vi "GUILaptop.vi"() -> ()   [LabVIEW 2016]
uses:
  Control/Fahrart.ctl
  Control/StreamCluster.ctl
  Control/GUICluster.ctl
panel:
  in  "Automatisch":bool
  out "stop 2":bool
  in  "Start":bool
  in  "Fahrzustand":T1
  in  "stop":bool
  in  "Geschwindigkeit multiplikator":dbl(knob)=0.039196582802747515 scale=0.0..1.0
  out "Linefollow-Array":bool[](array[boolean])
  out "Geschwindigkeit [m/s]":dbl(knob) scale=0.0..4.5
  out "Rundenzeit":T2
  out "schräg L":dbl format="%#_3g"
  out "schräge R":dbl format="%#_3g"
  out "hinten links":dbl
  out "Leistung [W]":dbl(graph)
  out "hinten rechts":dbl
  out "rechts":dbl format="%#_3g"
  out "links":dbl format="%#_3g"
  out "gerade L":dbl format="%#_3g"
  out "gerade R":dbl format="%#_3g"
  # "Minimum"
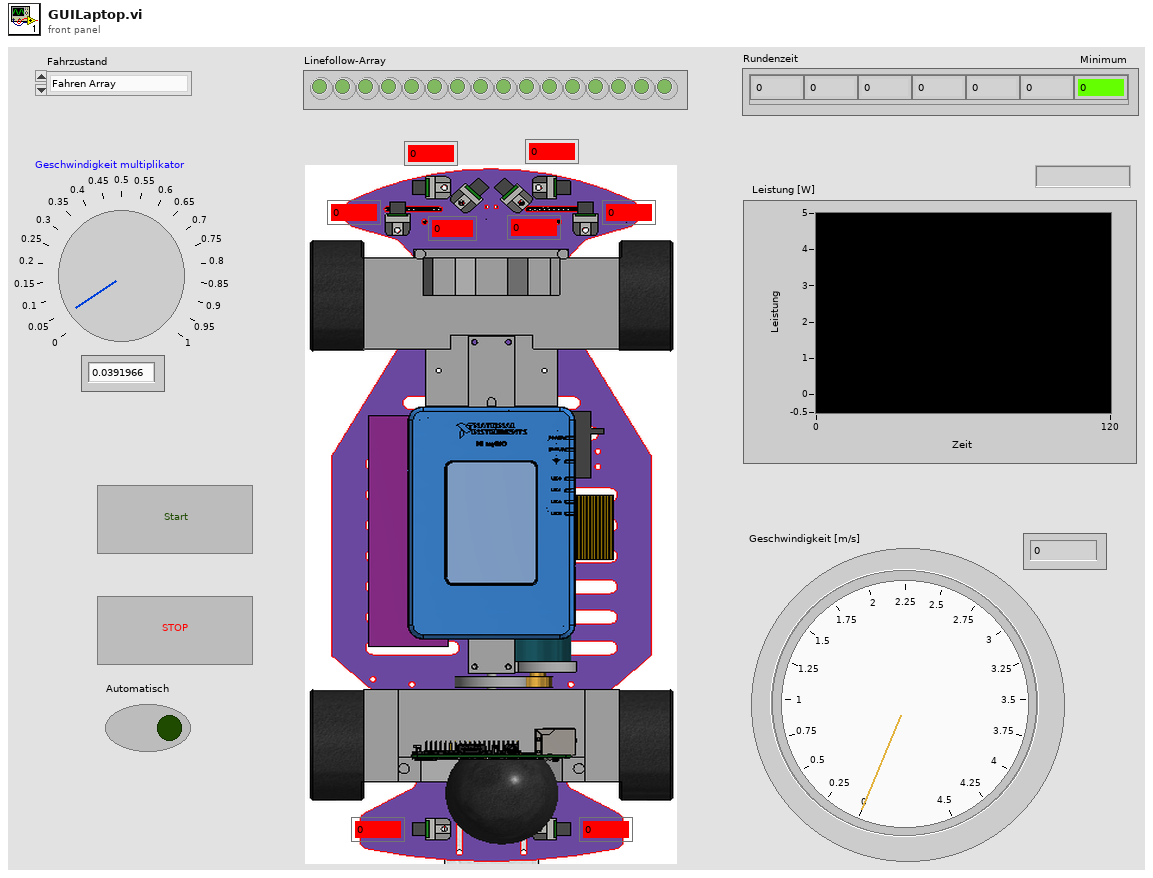
[diagram p1: front panel]
types:
  T1 = typedef "Fahrart.ctl" = enum16{"Fahren Array", "Folgen", "Überholen"}
  T2 = cluster{"Numeric":dbl, "Numeric 2":dbl, "Numeric 3":dbl, "Numeric 4":dbl, "Numeric 5":dbl, "Numeric 6":dbl, "Numeric 7":dbl}
  T3 = typedef "StreamCluster.ctl" = cluster{"IRSensoren":dbl[], "LineArray":bool[], "Rundenzeit":dbl[], "Drehzahl":dbl, "Leistung":dbl}
  T4 = typedef "GUICluster.ctl" = cluster{"Fahrart":T1, "Geschwindigkeitsmultiplikator":dbl, "Stop":bool, "Automatisch":bool}
  T5 = cluster{"Rundenzeit[0]":dbl, "Rundenzeit[1]":dbl, "Rundenzeit[2]":dbl, "Rundenzeit[3]":dbl, "Rundenzeit[4]":dbl, "Rundenzeit[5]":dbl, "Rundenzeit[6]":dbl}
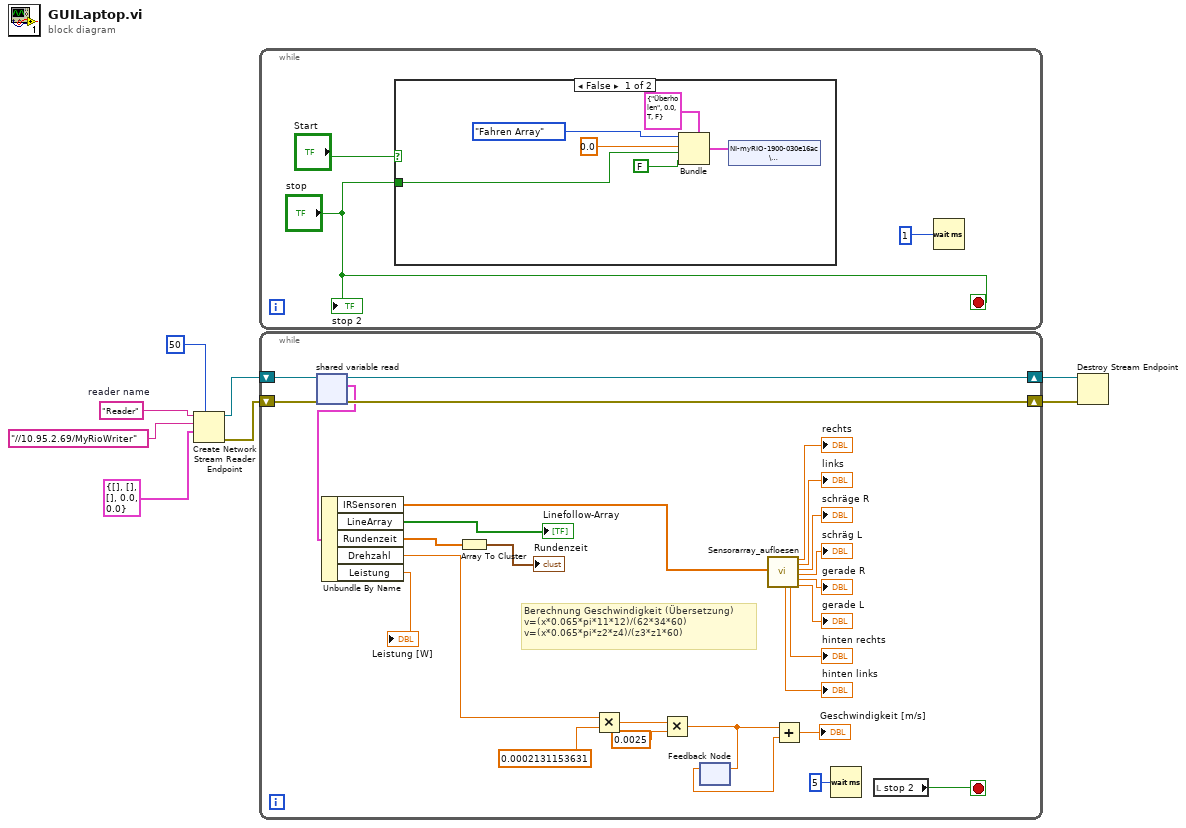
[diagram p0: block diagram]
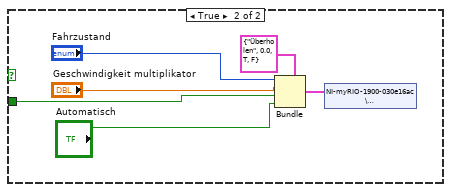
[diagram p2: hidden frame]
diagram:
  w4 = "Reader"  # reader name
  n1 = Create Network Stream Reader Endpoint(7:50 ("reader buffer size"), 9:T3 {"IRSensoren"=[], "LineArray"=[], "Rundenzeit"=[], "Drehzahl"=0.0, "Leistung"=0.0} ("Cluster"), 10:"//10.95.2.69/MyRioWriter" ("writer url"), 11:w4) -> (0:w7:errorcluster, 3:w8:refnum<k21>)  [unwired: 3 in]
  n2 = while {
    stop <- "stop" stop-if-true
    n3 = case shown="False" "Start" {
      tunnel: "stop" -> [w12 w18]
      frame False {
        n4 = Bundle(cluster=T4 {"Fahrart"=enum."Überholen", "Geschwindigkeitsmultiplikator"=0.0, "Stop"=TRUE, "Automatisch"=FALSE} ("Cluster"), "Fahrart"=Fahrart."Fahren Array" ("Enum"), "Geschwindigkeitsmultiplikator"=0.0, "Stop"=w12, "Automatisch"=FALSE ("Stop")) -> (w17:T4)
        n5 = shared-variable "NI-myRIO-1900-030e16ac\\GUICommunicationLibrary.lvlib\\GUIInput"(w17) -> ()  [unwired: 1 in, 1 out]
      }
      frame True {
        n6 = Bundle(cluster=T4 {"Fahrart"=enum."Überholen", "Geschwindigkeitsmultiplikator"=0.0, "Stop"=TRUE, "Automatisch"=FALSE} ("Cluster"), "Fahrart"="Fahrzustand", "Geschwindigkeitsmultiplikator"="Geschwindigkeit multiplikator", "Stop"=w18, "Automatisch"="Automatisch") -> (w21:T4)
        n7 = shared-variable "NI-myRIO-1900-030e16ac\\GUICommunicationLibrary.lvlib\\GUIInput"(w21) -> ()  [unwired: 1 in, 1 out]
      }
    }
    n8 = Wait (ms)(milliseconds to wait=u32 1) -> ()  [unwired: 1 out]
    "stop 2" <- "stop"
  }
  n9 = while {
    shift-right: [w40] -> w6
    shift-left: w8 -> [w42]
    shift-right: [w39] -> w5
    shift-left: w7 -> [w41]
    stop <- w43 stop-if-true
    # "Berechnung Geschwindigkeit (Übersetzung)\nv=(x*0.065*pi*11*12)/(62*34*60)\nv=(x*0.065*pi*z2*z4)/(z3*z1*60)"
    n10 = shared-variable-read(w42, w41) -> (w40:refnum<k21>, w39:errorcluster, w38:T3)  [unwired: 1 in, 1 out]
    n11 = Unbundle By Name(w38) -> ("IRSensoren"=w32:dbl[], "LineArray"=→"Linefollow-Array":bool[], "Rundenzeit"=w35:dbl[], "Drehzahl"=w37:dbl, "Leistung"=→"Leistung [W]":dbl)
    n12 = Array To Cluster(array=w35) -> (cluster=→"Rundenzeit":T5)
    n13 = Multiply(x=w37, y=0.0002131153631) -> (x*y=w49:dbl)
    n14 = Multiply(x=w49, y=0.0025) -> (x*y=w45:dbl)
    n15 = feedback-in #1(w45) -> ()
    n16 = feedback #1() -> (w46:dbl)  [unwired: 1 in]
    n17 = call "Sensorarray_aufloesen.vi"("Array"=w32) -> ("hinten links"=→"hinten links":dbl, "hinten rechts"=→"hinten rechts":dbl, 14:→"rechts":dbl, "vorne links"=→"links":dbl, "schräg rechts"=→"schräge R":dbl, "schräg links"=→"schräg L":dbl, "gerade rechts"=→"gerade R":dbl, "gerade links"=→"gerade L":dbl)  [unwired: 11 in]
    n18 = Add(x=w45, y=w46) -> (x+y=→"Geschwindigkeit [m/s]":dbl)
    n19 = Wait (ms)(milliseconds to wait=u32 5) -> ()  [unwired: 1 out]
    n20 = local read "stop 2"() -> (w43:bool)
  }
  n21 = Destroy Stream Endpoint(8:w5, 11:w6) -> ()  [unwired: 1 out]
